vi "Load Sequence from XML.vi"(8 "error in (no error)":errorcluster, 11 "Sequence Conditions In":T1 {"Sequence Controller"."Valve" items=["None", "LOX Press", "LOX Purge", "LOX Vent", "LOX Iso", "LOX Main", "LOX Bleed", "*open*", "Fuel Press", "Fuel Purge", "Fuel Vent", "Fuel Iso", "Fuel Main", "Film Cooling", "*open*", "Ignition"]}) -> (0 "error out":errorcluster, 3 "Sequence Conditions Out":T1 {"Sequence Controller"."Valve" items=["None", "LOX Press", "LOX Purge", "LOX Vent", "LOX Iso", "LOX Main", "LOX Bleed", "*open*", "Fuel Press", "Fuel Purge", "Fuel Vent", "Fuel Iso", "Fuel Main", "Film Cooling", "*open*", "Ignition"]})   [LabVIEW 2024]
doc: "Attempts to load previous user specified settings from an XML file.\n\nThis VI will not generate an error. If a suitable XML file can't be loaded and parsed then it will simply return the default settings."
uses:
  Sequence Structure.ctl
  <vilib>/Utility/xml.llb/Read From XML File(string).vi
  <vilib>/Utility/xml.llb/Write to XML File(string).vi
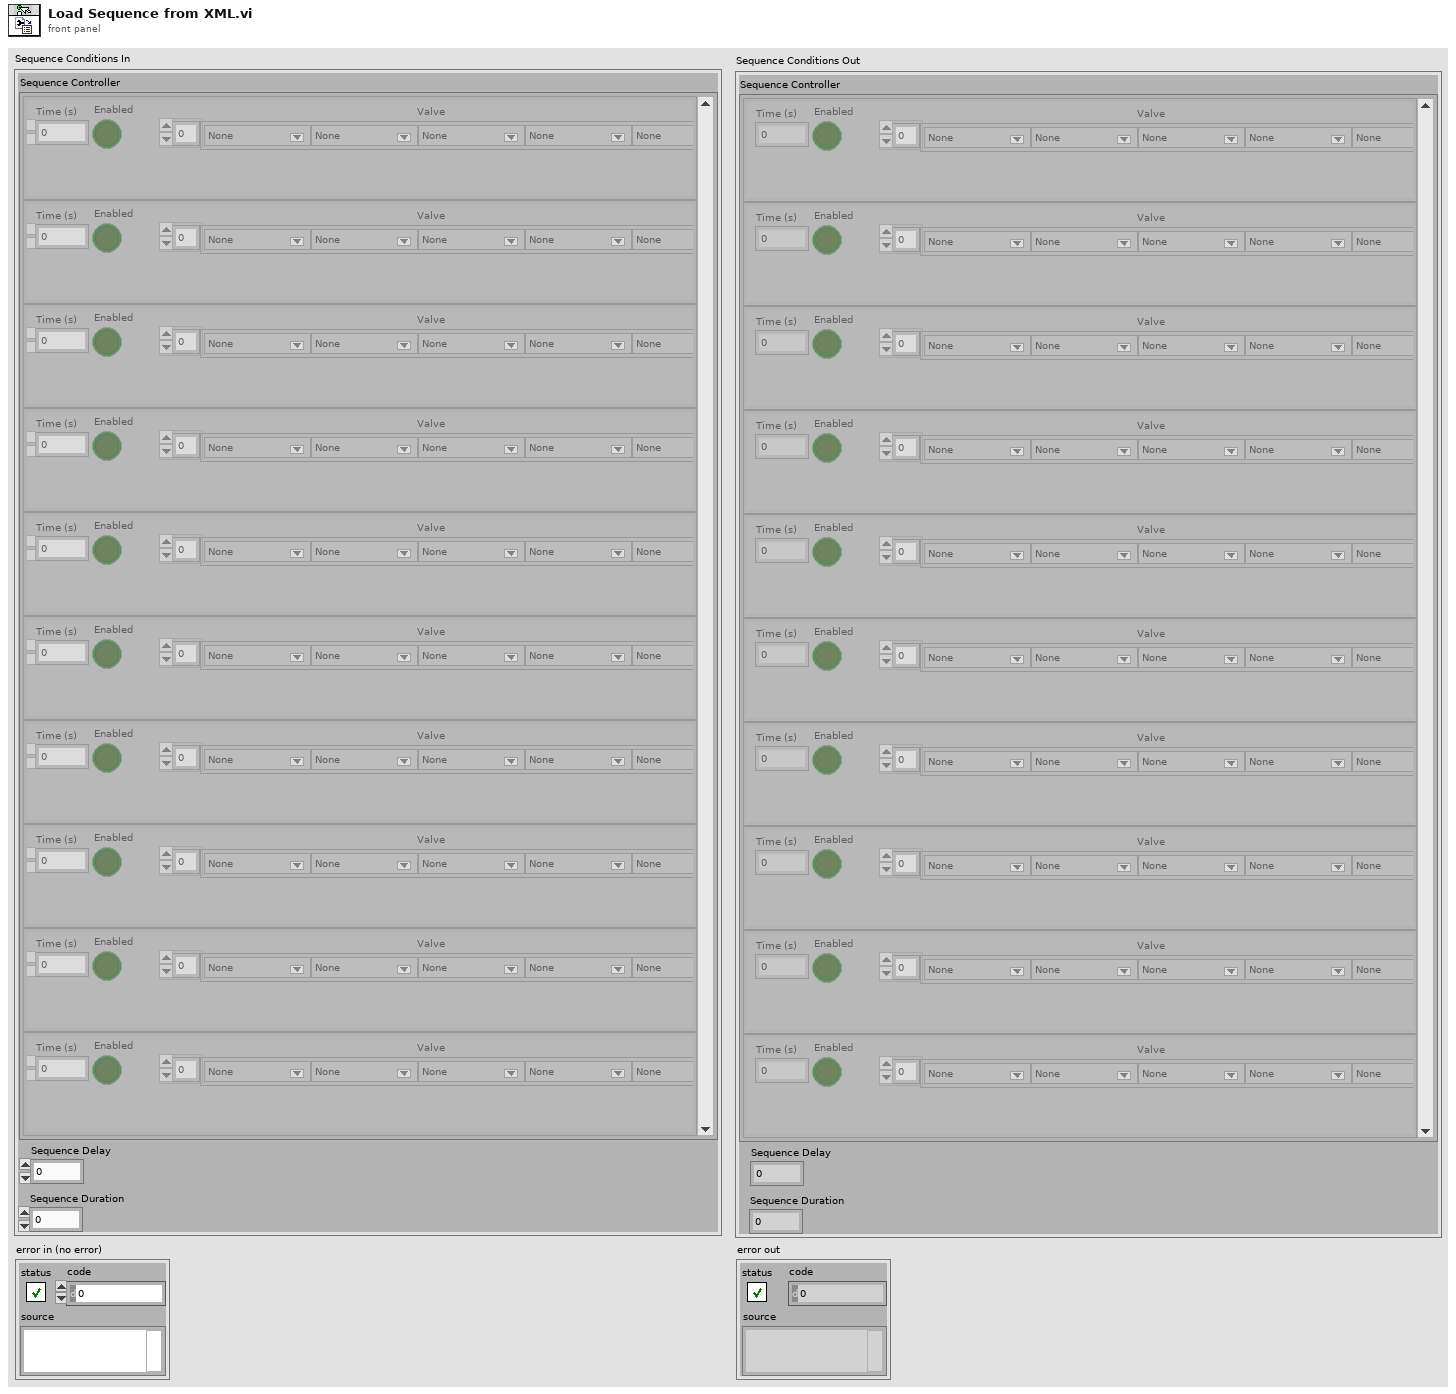
[diagram p1: front panel]
types:
  T1 = typedef "Sequence Structure.ctl" = cluster{"Sequence Controller":cluster{"Time (s)":dbl, "Enabled":bool, "Valve":u16[]}[], "Sequence Delay":dbl, "Sequence Duration":dbl}
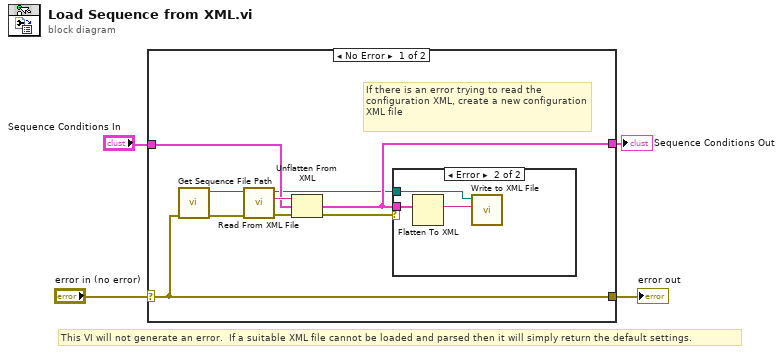
[diagram p0: block diagram]
diagram:
  # "This VI will not generate an error.  If a suitable XML file cannot be loaded and parsed then it will simply return the default settings."
  n1 = case shown="No Error" "error in (no error)" {
    selector: "error in (no error)" -> [w5 w17]
    tunnel: [w5 w17] -> w3
    tunnel: "Sequence Conditions In" -> [w9 w16]
    tunnel: [w8 w16] -> w1
    frame No Error {
      # "If there is an error trying to read the configuration XML, create a new configuration XML file"
      n2 = call "Get Sequence File Path.vi"("error in (no error)"=w5) -> ("error out"=w6:errorcluster, "XML File Path"=w7:path)  [unwired: 9 in]
      n3 = call-poly <vilib>:"Read From XML File.vi"("error in (no error)"=w6, "XML File Path"=w7) -> ("error out"=w11:errorcluster, "XML Elements"=w12:string)  [unwired: 7 in, 1 out]
      n4 = Unflatten From XML(xml string=w12, type=w9, error in (no error)=w11) -> (value=w8:T1, error out=w10:errorcluster)
      n5 = case shown="Error" w10 {
        tunnel: w8 -> [_ w15]
        tunnel: w7 -> [_ w13]
        frame No Error {
        }
        frame Error {
          n6 = Flatten To XML(6:w15) -> (2:w14:string)
          n7 = call-poly <vilib>:"Write to XML File.vi"("XML Input"=w14, "XML File Path"=w13) -> ()  [unwired: 7 in, 3 out]
        }
      }
    }
    frame Error {
    }
  }
  "error out" <- w3
  "Sequence Conditions Out" <- w1
